vi "UART_B_ver2.vi"(0 "VISA Refnum in":refnum<visa-resource-name>, 1 "Señal_2":dbl, 2 "Señal_1":dbl, 3 "VISA Configuration":T1 {"termination char\n(0xA = '\\n' = LF)" format="%.0x"; "flow control (0:none)" items=["None", "XON/XOFF", "RTS/CTS", "XON/XOFF & RTS/CTS", "DTR/DSR", "XON/XOFF & DTR/DSR"]; "stop bits (10: 1 bit)" items=["1.0"=10, "1.5"=15, "2.0"=20]; "data bits (8)" min=5 max=8 step=1}, 4 "Señal_5":dbl, 5 "Señal_4":dbl, 7 "error in (no error)":errorcluster, 8 "Señal_3":dbl) -> (12 "Characters Read":string, 14 "US_1":string, 16 "Sensor_1":dbl, 17 "Trama Recibida":string, 18 "Sensor_2":dbl, 20 "US_2":string, 21 "Trama de envio":string, 22 "Sensor_3":dbl, 23 "US_3":string, 27 "error out":errorcluster)   [LabVIEW 2019]
uses:
  <vilib>/myRIO/Instrument Drivers/Onboard IO/UART/typedef/VISA Configuration.ctl
  <vilib>/Instr/_visa.llb/VISA Configure Serial Port (Instr).vi
  <vilib>/myRIO/Express VI/Onboard IO/UART/UART Express VI.xnode
  <vilib>/myRIO/Instrument Drivers/Onboard IO/UART/UART.lvlib
panel:
  out "Sensor_5":dbl
  out "US_3 3":string
  out "Sensor_4":dbl
  out "US_3 2":string
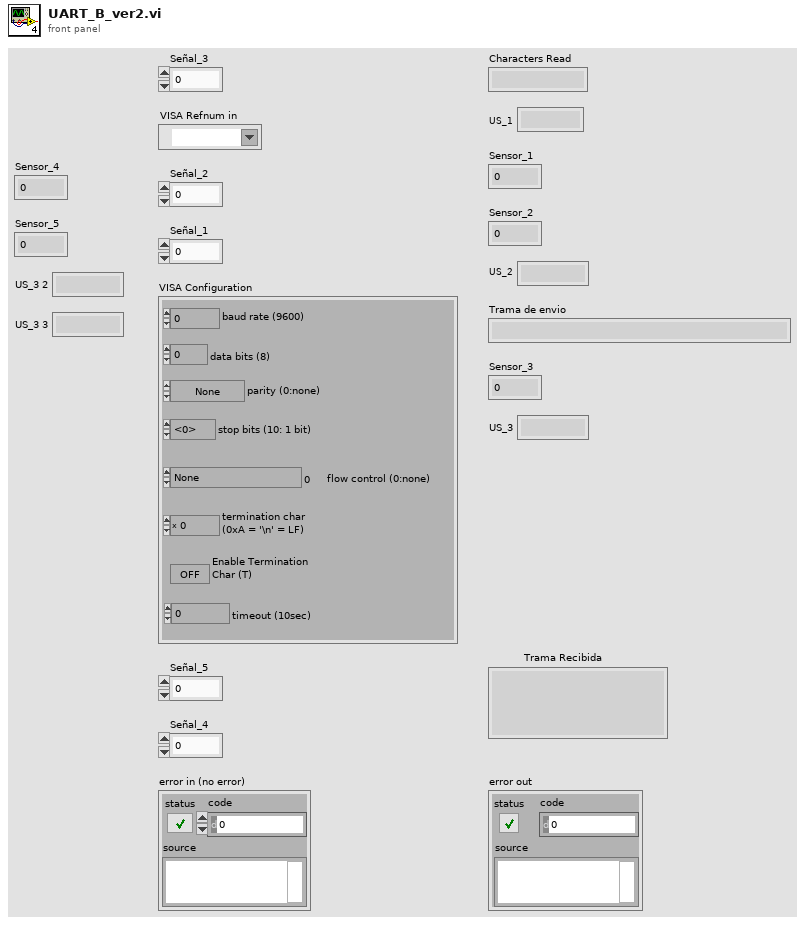
[diagram p1: front panel]
types:
  T1 = typedef "UART.lvlib/VISA Configuration.ctl" = cluster{"baud rate (9600)":u32, "data bits (8)":u16, "parity (0:none)":enum16{"None", "Odd", "Even", "Mark", "Space"}, "stop bits (10: 1 bit)":u16, "flow control (0:none)":u16, "termination char\n(0xA = '\\n' = LF) ":u8, "Enable Termination\nChar (T)":bool, "timeout (10sec)":u32}
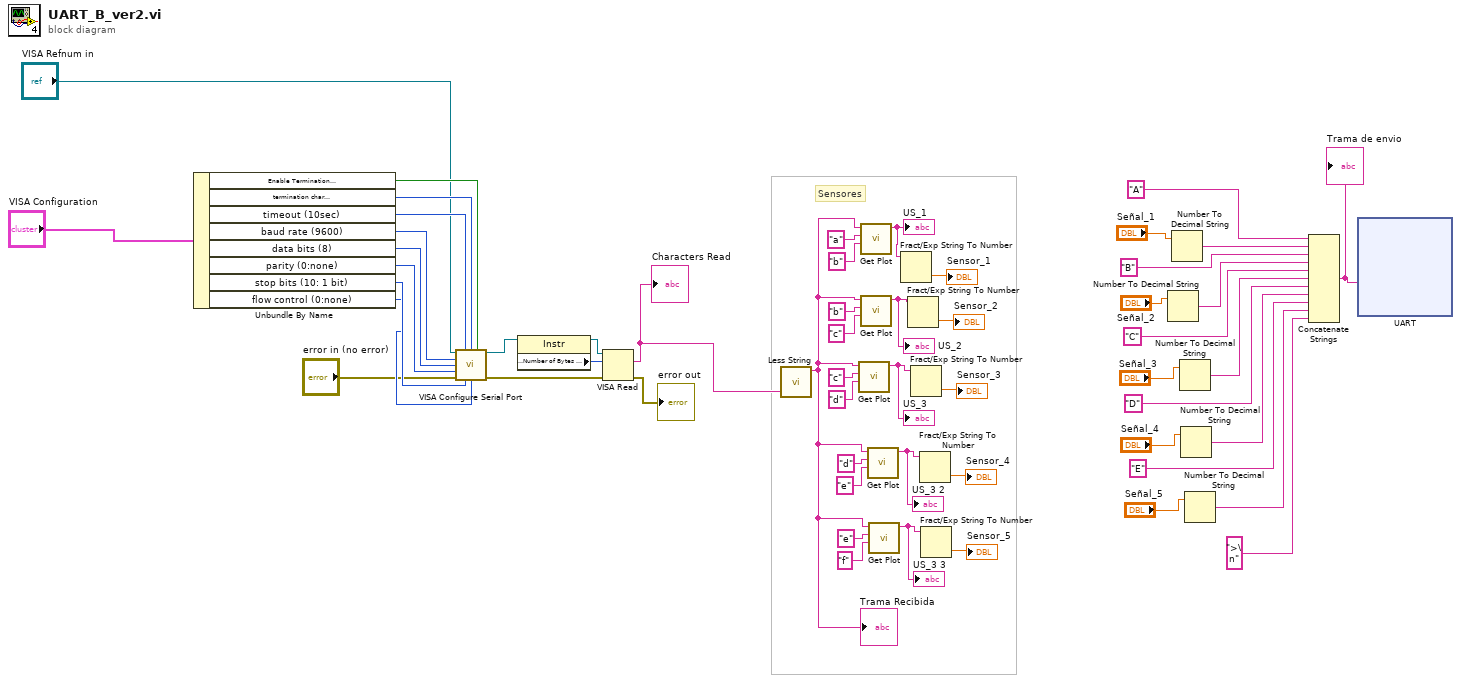
[diagram p0: block diagram]
diagram:
  # "Sensores"
  n1 = Unbundle By Name("VISA Configuration") -> ("Enable Termination\nChar (T)"=w13:bool, "termination char\n(0xA = '\\n' = LF)"=w14:u8, "timeout (10sec)"=w15:u32, "baud rate (9600)"=w20:u32, "data bits (8)"=w19:u16, "parity (0:none)"=w18:enum16{"None", "Odd", "Even", "Mark", "Space"}, "stop bits (10: 1 bit)"=w17:u16, "flow control (0:none)"=w16:u16)
  n2 = call-poly "VISA Configure Serial Port"("VISA resource name"="VISA Refnum in", "timeout (10sec)"=w15, "termination char\n(0xA = '\\n' = LF)"=w14, "Enable Termination\nChar (T)"=w13, "baud rate (9600)"=w20, "data bits (8)"=w19, "parity (0:none)"=w18, "error in (no error)"="error in (no error)", "stop bits (10: 1 bit)"=w17, "flow control (0:none)"=w16) -> ("VISA resource name out"=w21:refnum<visa-resource-name>, "error out"=w22:errorcluster)  [unwired: 4 in]
  n3 = property class="Instr"(reference=w21) -> (reference out=w29:refnum<visa-resource-name>, "Serial Settings:Number of Bytes at Serial Port"=w30:u32)  [unwired: 1 in, 1 out]
  n4 = VISA Read(VISA resource name=w29, byte count=w30, error in (no error)=w22) -> (read buffer=w31:string, error out=→"error out":errorcluster)  [unwired: 2 out]
  "Characters Read" <- w31
  n5 = call "Less String.vi"("Input String"=w31) -> ("Out String"=w1:string)  [unwired: 10 in]
  "Trama Recibida" <- w1
  n6 = call "Get Plot.vi"("Stop"="d", "Start"="c", "Input String"=w1) -> ("Out String"=w39:string)  [unwired: 8 in]
  "US_3" <- w39
  n7 = call "Get Plot.vi"("Stop"="b", "Start"="a", "Input String"=w1) -> ("Out String"=w34:string)  [unwired: 8 in]
  "US_1" <- w34
  n8 = call "Get Plot.vi"("Stop"="c", "Start"="b", "Input String"=w1) -> ("Out String"=w38:string)  [unwired: 8 in]
  "US_2" <- w38
  n9 = call "Get Plot.vi"("Stop"="e", "Start"="d", "Input String"=w1) -> ("Out String"=w5:string)  [unwired: 8 in]
  "US_3 2" <- w5
  n10 = call "Get Plot.vi"("Stop"="f", "Start"="e", "Input String"=w1) -> ("Out String"=w9:string)  [unwired: 8 in]
  "US_3 3" <- w9
  n11 = Fract/Exp String To Number(string=w34) -> (number=→"Sensor_1":dbl)  [unwired: 3 in, 1 out]
  n12 = Fract/Exp String To Number(string=w38) -> (number=→"Sensor_2":dbl)  [unwired: 3 in, 1 out]
  n13 = Fract/Exp String To Number(string=w39) -> (number=→"Sensor_3":dbl)  [unwired: 3 in, 1 out]
  n14 = Fract/Exp String To Number(string=w5) -> (number=→"Sensor_4":dbl)  [unwired: 3 in, 1 out]
  n15 = Fract/Exp String To Number(string=w9) -> (number=→"Sensor_5":dbl)  [unwired: 3 in, 1 out]
  n16 = Number To Decimal String(number="Señal_2") -> (decimal integer string=w42:string)  [unwired: 1 in]
  n17 = Number To Decimal String(number="Señal_1") -> (decimal integer string=w40:string)  [unwired: 1 in]
  n18 = Number To Decimal String(number="Señal_3") -> (decimal integer string=w44:string)  [unwired: 1 in]
  n19 = Number To Decimal String(number="Señal_4") -> (decimal integer string=w52:string)  [unwired: 1 in]
  n20 = Number To Decimal String(number="Señal_5") -> (decimal integer string=w54:string)  [unwired: 1 in]
  n21 = Concatenate Strings("A" ("string"), w40, "B" ("string"), w42, "C" ("string"), w44, "D" ("string"), w52, "E" ("string"), w54, ">\n" ("string")) -> (w33:string)
  "Trama de envio" <- w33
  n22 = xnode "UART"("Characters to Write"=w33) -> ()  [unwired: 1 in, 2 out]
